vi "test Receive Message.vi"(8 "error in (no error)":errorcluster, 11 "TestCase in":refnum<class "Test Network Stream Transmission.lvclass">) -> (0 "error out":errorcluster, 3 "TestCase out":refnum<class "Test Network Stream Transmission.lvclass">)   [LabVIEW 2020, in "Test Network Stream Transmission.lvclass"]
uses:
  Test Network Stream Transmission.lvclass
  <vilib>/addons/_JKI Toolkits/VI Tester/TestCase.llb/TestCase.lvclass
  Source/Protocols/Network Stream Strategy/Network Stream Initiator/Network Stream Initiator.lvclass
  <vilib>/ActorFramework/LastAck/Last Ack.lvclass
  Source/Abstract Classes/Cipher/Cipher.lvclass
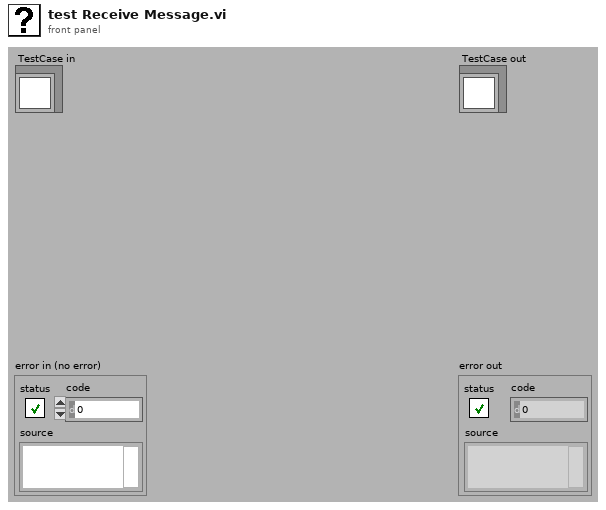
[diagram p1: front panel]
types:
  T1 = cluster{"Last Ack":refnum<class "Last Ack.lvclass">, "priority":i32}
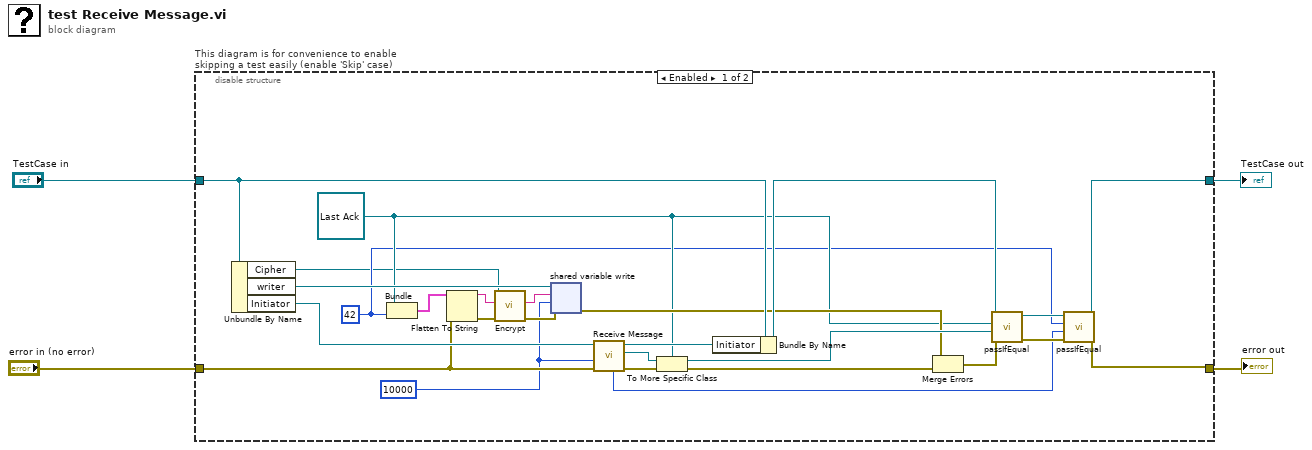
[diagram p0: block diagram]
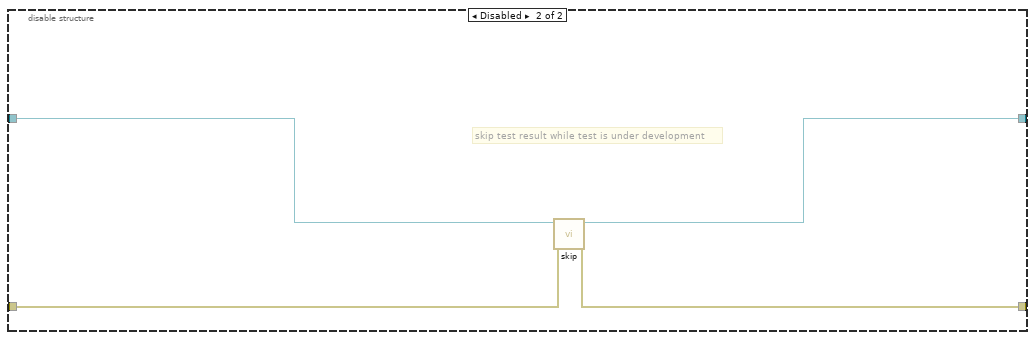
[diagram p2: hidden frame]
diagram:
  n1 = disable-structure "This diagram is for convenience to enable skipping a test easily (enable 'Skip' case)" shown="Enabled" {
    disable-tunnel: "TestCase in" -> [w24 w34]
    disable-tunnel: [w15 w32] -> w1
    disable-tunnel: [w13 w33] -> w3
    disable-tunnel: "error in (no error)" -> [w28 w31]
    frame Enabled {
      w12 = 42 ("priority")
      w7 = 10000 ("timeout ms (-1)")
      w17 = refnum<class "Last Ack.lvclass"> refnum ("Last Ack")
      n2 = Unbundle By Name(w24) -> ("Cipher"=w5:refnum<class "Cipher.lvclass">, "writer"=w30:refnum<k21>, "Initiator"=w29:refnum<class "Network Stream Initiator.lvclass">)
      n3 = Bundle("Last Ack"=w17, "priority"=w12) -> (w18:T1)  [unwired: 1 in]
      n4 = Flatten To String(anything=w18, error in (no error)=w28) -> (data string=w9:string, error out=w10:errorcluster)  [unwired: 2 in, 1 out]
      n5 = call-dynamic "Encrypt.vi"("error in (no error)"=w10, "Plaintext"=w9, "Cipher in"=w5) -> ("error out"=w8:errorcluster, "Cyphertext"=w6:string)  [unwired: 6 in, 1 out]
      n6 = shared-variable-write(w30, w8, w6, w7) -> (w19:errorcluster)  [unwired: 2 out]
      n7 = call-dynamic "Receive Message.vi"("error in (no error)"=w28, "timeout ms (-1)"=w7, "Network Stream in"=w29) -> ("error out"=w26:errorcluster, "Message"=w27:refnum<class "Message.lvclass">, "Network Stream out"=w22:refnum<class "Network Stream Initiator.lvclass">, "priority"=w11:i32)  [unwired: 4 in, 1 out]
      n8 = To More Specific Class(target class=w17, reference=w27, error in=w26) -> (specific class reference=w21:refnum<class "Last Ack.lvclass">, error out=w25:errorcluster)
      n9 = Bundle By Name(cluster=w24, "Initiator"=w22) -> (w23:refnum<class "Test Network Stream Transmission.lvclass">)
      n10 = Merge Errors(w19, w25) -> (w20:errorcluster)
      n11 = call-dynamic "passIfEqual.vi"("error in (no error)"=w20, "y"=w21, "x"=w17, "TestCase in"=w23) -> ("error out"=w14:errorcluster, "TestCase out"=w16:refnum<class "Test Network Stream Transmission.lvclass">)  [unwired: 6 in]
      n12 = call-dynamic "passIfEqual.vi"("error in (no error)"=w14, "y"=w11, "x"=w12, "TestCase in"=w16) -> ("error out"=w13:errorcluster, "TestCase out"=w15:refnum<class "Test Network Stream Transmission.lvclass">)  [unwired: 6 in]
    }
    frame Disabled {
      # "skip test result while test is under development"
      n13 = call <vilib>:"skip.vi"("error in (no error)"=w31, "TestCase in"=w34) -> ("error out"=w33:errorcluster, "TestCase out"=w32:refnum<class "Test Network Stream Transmission.lvclass">)  [unwired: 8 in]
    }
  }
  "error out" <- w3
  "TestCase out" <- w1
